vi "SSC DCPower Get Aperture Times in Seconds.vi"(0 "DCPower SSC in":T1[](array[typedef]), 11 "error in":errorcluster) -> (4 "DCPower SSC out":T1[](array[typedef]), 6 "Actual Aperture Times (s)":dbl[](array[numeric]) format="%#_6p", 8 "Maximum Aperture Time (s)":dbl format="%#_6p", 15 "error out":errorcluster)   [LabVIEW 2019]
doc: "This VI gets the measurement aperture time of the sessions in seconds (if it was set in units of PLCs, it converts it to seconds)."
uses:
  SSC DCPower.ctl
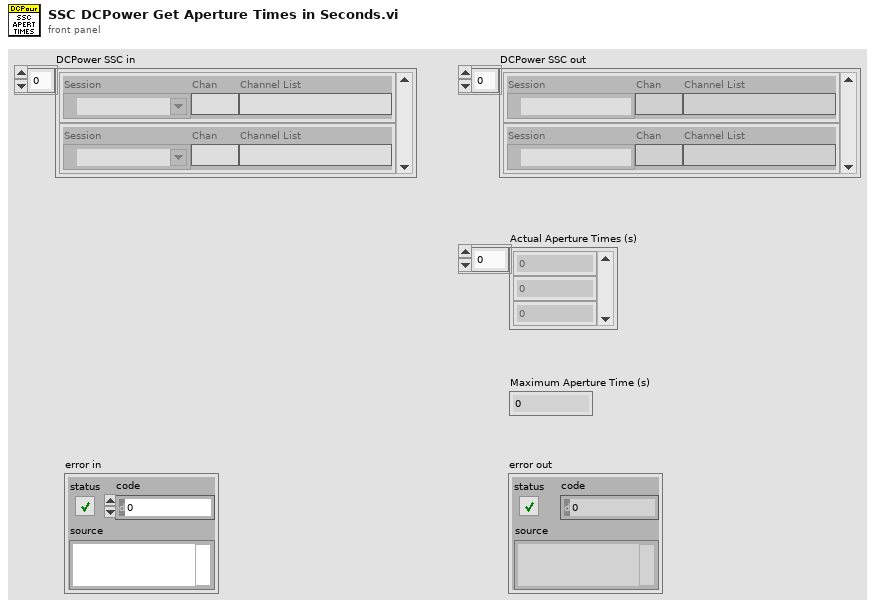
[diagram p1: front panel]
types:
  T1 = typedef "SSC DCPower.ctl" = cluster{"Session":refnum<k15>, "Chan":string, "Channel List":string}
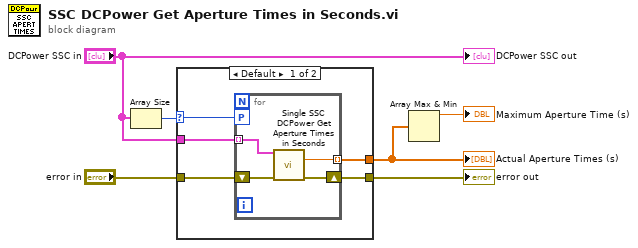
[diagram p0: block diagram]
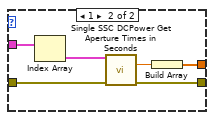
[diagram p2: hidden frame]
diagram:
  n1 = Array Size(array="DCPower SSC in") -> (size(s)=w3:i32)
  n2 = case shown="Default" w3 {
    selector: w3 -> [w9 _]
    tunnel: "error in" -> [w11 w21]
    tunnel: [w10 w20] -> w5
    tunnel: "DCPower SSC in" -> [w8 w19]
    tunnel: [w7 w16] -> w1
    frame Default {
      n3 = for {
        tunnel: w8 -> [w14] mode=indexing
        workers-P: w9 -> [_]
        shift-right: [w13] -> w10
        shift-left: w11 -> [w15]
        tunnel: [w12] -> w7 mode=indexing
        n4 = call "Single SSC DCPower Get Aperture Times in Seconds.vi"("DCPower SSC in"=w14, "error in"=w15) -> ("Actual Aperture Times (s)"=w12:dbl, "error out"=w13:errorcluster)  [unwired: 11 in, 1 out]
      }
    }
    frame 1 {
      n5 = Index Array(array=w19) -> (element=w17:T1)  [unwired: 1 in]
      n6 = call "Single SSC DCPower Get Aperture Times in Seconds.vi"("DCPower SSC in"=w17, "error in"=w21) -> ("Actual Aperture Times (s)"=w18:dbl, "error out"=w20:errorcluster)  [unwired: 11 in, 1 out]
      n7 = Build Array(w18) -> (w16:dbl[])
    }
  }
  "Actual Aperture Times (s)" <- w1
  "error out" <- w5
  n8 = Array Max & Min(array=w1) -> (max value=→"Maximum Aperture Time (s)":dbl)  [unwired: 3 out]
  "DCPower SSC out" <- "DCPower SSC in"
